vi "Z.关闭饼状图.vi"(8 "error in":errorcluster, 11 "Module ID":i32=-1) -> (0 "error out":errorcluster)   [LabVIEW 2020, in "PichartInterface.lvlib"]
uses:
  PichartInterface.lvlib
  <vilib>/DD/DDToolsVIPM/PieChartInterface/PieChart.lvlibp
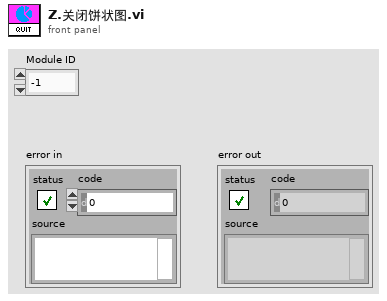
[diagram p1: front panel]
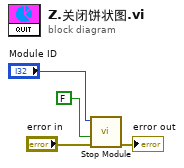
[diagram p0: block diagram]
diagram:
  n1 = call <vilib>:"Stop Module.vi"("error in"="error in", "Wait for Module to stop? (F)"=FALSE, "Module ID"="Module ID") -> ("error out"=→"error out":errorcluster)  [unwired: 8 in]
